vi "Initialize.vi"(8 "error in (no error)":errorcluster, 11 "ATM Data":T1={"UI Refs"={"Right Buttons"=refnum, "Left Buttons"=refnum, "User Input"=refnum, "ATM Messages"=refnum, "Left Menu"=refnum, "Right Menu"=refnum, "Enter"=refnum}, "Map"={}, "Login Valid?"=FALSE, "Queue Message"=refnum, "State"=enum."None", "User"={"Pin"="", "First Name"="", "Last Name"="", "Balance"=0.0, "Login Valid?"=FALSE}, "Main States"={"Message"="Initialize", "Data"=variant}}) -> (0 "error out":errorcluster, 3 "ATM Data Out":T1={"UI Refs"={"Right Buttons"=refnum, "Left Buttons"=refnum, "User Input"=refnum, "ATM Messages"=refnum, "Left Menu"=refnum, "Right Menu"=refnum, "Enter"=refnum}, "Map"={}, "Login Valid?"=FALSE, "Queue Message"=refnum, "State"=enum."None", "User"={"Pin"="", "First Name"="", "Last Name"="", "Balance"=0.0, "Login Valid?"=FALSE}, "Main States"={"Message"="Initialize", "Data"=variant}})   [LabVIEW 2020, in "ATM Machine.lvlib"]
uses:
  ATM Machine.lvlib
  Cluster - ATM Machine Data.ctl
  Cluster - Message Cluster.ctl
  Enum - ATM States.ctl
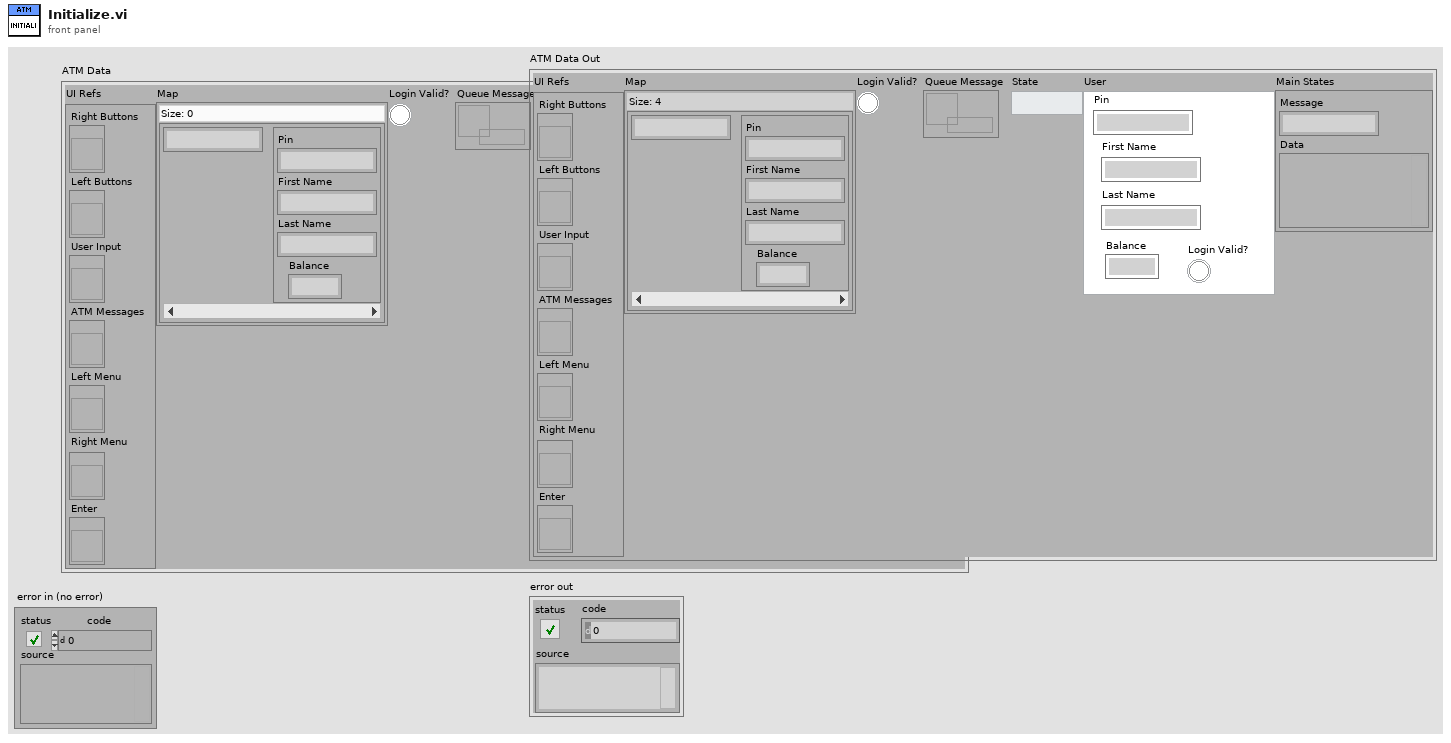
[diagram p1: front panel]
types:
  T1 = typedef "ATM Machine.lvlib/Cluster - ATM Machine Data.ctl" = cluster{"UI Refs":cluster{"Right Buttons":refnum<vi>, "Left Buttons":refnum<vi>, "User Input":refnum<vi>, "ATM Messages":refnum<vi>, "Left Menu":refnum<vi>, "Right Menu":refnum<vi>, "Enter":refnum<vi>}, "Map":map{string, cluster{"Pin":string, "First Name":string, "Last Name":string, "Balance":dbl}}, "Login Valid?":bool, "Queue Message":refnum<queue>, "State":T2, "User":cluster{"Pin":string, "First Name":string, "Last Name":string, "Balance":dbl, "Login Valid?":bool}, "Main States":cluster{"Message":string, "Data":variant}}
  T2 = typedef "ATM Machine.lvlib/Enum - ATM States.ctl" = enum16{"None", "Deposit", "Withdraw", "Card Inserted", "Balance Inquiry", "Return Card and Terminate", "Fast Cash"}
  T3 = enum8{"Enabled", "Disabled", "Disabled and Grayed Out"}
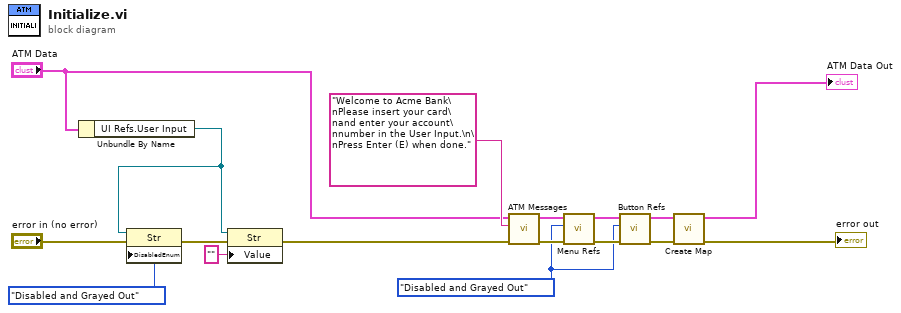
[diagram p0: block diagram]
diagram:
  w8 = T3."Disabled and Grayed Out" ("Disabled 2")
  n1 = Unbundle By Name("ATM Data") -> ("UI Refs.User Input"=w2:refnum<vi>)
  n2 = property class="Str"(reference=w2, error in="error in (no error)", "DisabledEnum"=T3."Disabled and Grayed Out" ("Disabled")) -> (error out=w3:errorcluster)  [unwired: 1 out]
  n3 = property class="Str"(reference=w2, error in=w3, "Value"="") -> (error out=w6:errorcluster)  [unwired: 1 out]
  n4 = call "ATM Messages.vi"("error in"=w6, "ATM Message"="Welcome to Acme Bank\nPlease insert your card\nand enter your account\nnumber in the User Input.\n\nPress Enter (E) when done.", "ATM Data"="ATM Data") -> ("error out"=w15:errorcluster, "ATM Data Out"=w14:T1)  [unwired: 7 in]
  n5 = call "Menu Refs.vi"("error in"=w15, "Disabled 2"=w8, "ATM Data"=w14) -> ("error out"=w17:errorcluster, "ATM Data Out"=w16:T1)  [unwired: 7 in]
  n6 = call "Button Refs.vi"("error in"=w17, "Disabled"=w8, "ATM Data"=w16) -> ("error out"=w12:errorcluster, "ATM Data Out"=w10:T1)  [unwired: 7 in]
  n7 = call "Create Map.vi"("error in (no error)"=w12, "ATM Data"=w10) -> ("error out"=→"error out":errorcluster, "ATM Data Out"=→"ATM Data Out":T1)  [unwired: 8 in]
